vi "convert_string_to_double.vi"(3 "default (0)":dbl, 4 "String in":string) -> (1 "double value out":dbl)   [LabVIEW 2014, in "rszvl_rsidr_core.lvlib"]
uses:
  rszvl_rsidr_core.lvlib
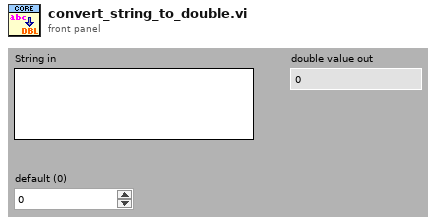
[diagram p1: front panel]
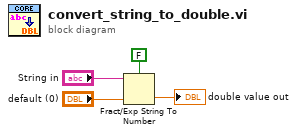
[diagram p0: block diagram]
diagram:
  n1 = Fract/Exp String To Number(use system decimal point (T)=FALSE, string="String in", default (0 dbl)="default (0)") -> (number=→"double value out":dbl)  [unwired: 1 in, 1 out]
